vi "Calc P4.vi"(9 "Bottom":T1, 10 "Middle":T1, 11 "Top":T1) -> (3 "Point 4":T1)   [LabVIEW 2022 SP3, in "Raster.lvlib"]
uses:
  Point 2D.ctl
  Raster.lvlib
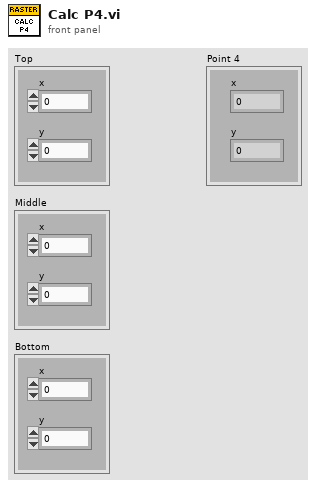
[diagram p1: front panel]
types:
  T1 = typedef "Raster.lvlib/Point 2D.ctl" = cluster{"x":i32, "y":i32}
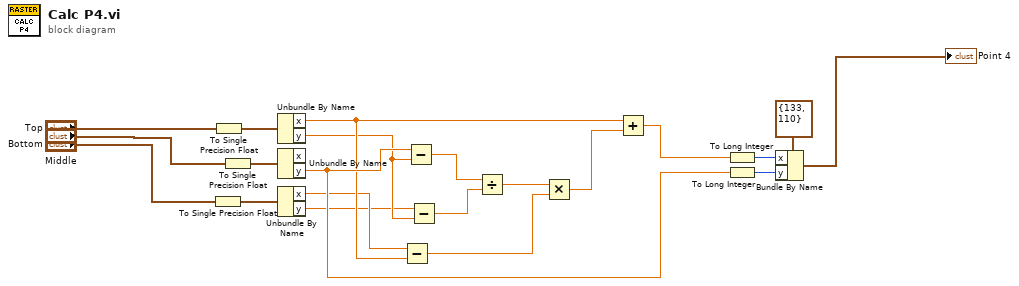
[diagram p0: block diagram]
diagram:
  n1 = To Single Precision Float(number="Bottom") -> (single precision float=w4:cluster{"x":sgl, "y":sgl})
  n2 = To Single Precision Float(number="Top") -> (single precision float=w5:cluster{"x":sgl, "y":sgl})
  n3 = To Single Precision Float(number="Middle") -> (single precision float=w21:cluster{"x":sgl, "y":sgl})
  n4 = Unbundle By Name(w5) -> ("x"=w7:sgl, "y"=w2:sgl)
  n5 = Unbundle By Name(w21) -> ("y"=w15:sgl)  [unwired: 1 out]
  n6 = Unbundle By Name(w4) -> ("x"=w6:sgl, "y"=w1:sgl)
  n7 = Subtract(x=w6, y=w7) -> (x-y=w10:sgl)
  n8 = Subtract(x=w15, y=w2) -> (x-y=w3:sgl)
  n9 = Subtract(x=w1, y=w2) -> (x-y=w8:sgl)
  n10 = Divide(x=w3, y=w8) -> (x/y=w9:sgl)
  n11 = Multiply(x=w9, y=w10) -> (x*y=w11:sgl)
  n12 = Add(x=w7, y=w11) -> (x+y=w13:sgl)
  n13 = To Long Integer(number=w13) -> (32bit integer=w14:i32)
  n14 = To Long Integer(number=w15) -> (32bit integer=w16:i32)
  n15 = Bundle By Name(cluster=T1 {"x"=133, "y"=110} ("Point 1"), "x"=w14, "y"=w16) -> (→"Point 4":T1)
